vi "run.vi"(8 "error in (no error)":errorcluster, 11 "GenericScanMode in":refnum<class "GenericImagingMode.lvclass">) -> (0 "error out":errorcluster, 3 "GenericScanMode out":refnum<class "GenericImagingMode.lvclass">)   [LabVIEW 2010, in "GenericImagingMode.lvclass"]
uses:
  GenericImagingMode.lvclass
  common/classes/GenericToplevelComponent/GenericToplevelComponent/common_trigger_enum.ctl
  common/classes/ErrorController/ErrorController/class_data.vi
  common/classes/ErrorController/ErrorController/ErrorController.lvclass
  common/classes/GenericToplevelComponent/GenericToplevelComponent/GenericToplevelComponent.lvclass
panel:
  # "Functionality not available..."
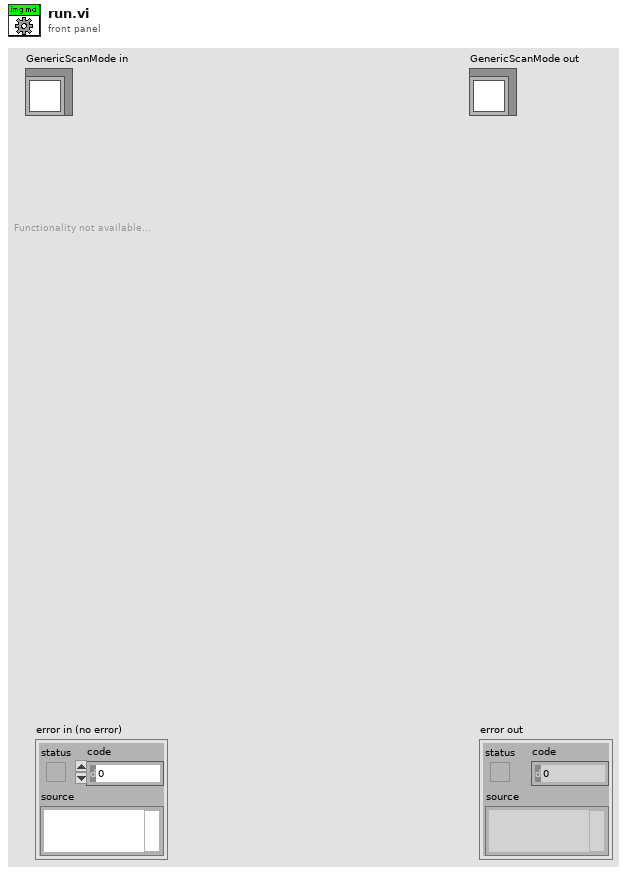
[diagram p1: front panel]
types:
  T1 = typedef "GenericToplevelComponent.lvclass/common_trigger_enum.ctl" = enum16{"NULL", "initialise", "terminate", "fetch command", "fetch data", "attach observer", "register as observer", "detach observer", "acknowledge", "start", "stop", "sweep started", "sweep finished", "experiment started", "experiment stopped"}
  T2 = typedef "main_trigger_enum.ctl" = enum16{"NULL", "initialise", "terminate", "start", "stop", "change objective", "change experimentController", "change imagingMode", "save notebook", "started saving", "finished saving", "expCtr ready", "expCtr missing", "imgMd ready", "imgMd missing", "scanHd ready", "scanHd missing", "DAQ ready", "DAQ missing", "imgAsm ready", "imgAsm missing", "dataColl ready", "dataColl missing", "display ready", "display missing", "analysr ready", "analysr missing", "instrmnt ready", "instrmnt missing", "stimltr ready", "stimltr missing", "stage ready", "stage missing"}
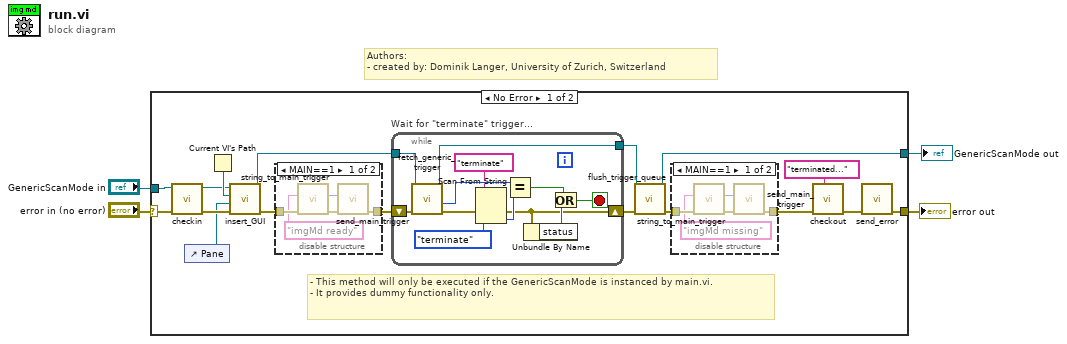
[diagram p0: block diagram]
diagram:
  # "Authors: \n- created by: Dominik Langer, University of Zurich, Switzerland"
  n1 = case shown="No Error" "error in (no error)" {
    selector: "error in (no error)" -> [w12 w47]
    tunnel: [w20 w47] -> w2
    tunnel: [w18 w46] -> w1
    tunnel: "GenericScanMode in" -> [w11 w46]
    frame No Error {
      # "- This method will only be executed if the GenericScanMode is instanced by main.vi.\n- It provides dummy functionality only."
      n2 = call-dynamic "checkin.vi"("error in (no error)"=w12, "GenericScanMode in"=w11) -> ("error out"=w10:errorcluster, "GenericScanMode out"=w9:refnum<class "GenericImagingMode.lvclass">)  [unwired: 8 in]
      n3 = control-ref of="Pane"() -> (w5:refnum<vi>)
      n4 = Current VI's Path() -> (path=w21:path)
      n5 = call-dynamic "insert_GUI.vi"("error in (no error)"=w10, "Pane"=w5, "VI path"=w21, "GenericComponent in"=w9) -> ("error out"=w14:errorcluster, "GenericComponent out"=w16:refnum<class "GenericImagingMode.lvclass">)  [unwired: 6 in]
      n6 = disable-structure shown="MAIN==1" {
        disable-tunnel: [w26 w27] -> w13
        disable-tunnel: w14 -> [w25 w27]
        frame condition #0 {
          n7 = call "string_to_main_trigger.vi"("error in (no error)"=w25, "trigger string"="imgMd ready") -> ("error out"=w24:errorcluster, "main trigger"=w23:T2)  [unwired: 8 in]
          n8 = call "send_main_trigger.vi"("error in (no error)"=w24, "trigger"=w23) -> ("error out"=w26:errorcluster)  [unwired: 9 in]
        }
        frame condition #1 (active) {
        }
      }
      n9 = while "Wait for \"terminate\" trigger..." {
        tunnel: w16 -> [w42]
        tunnel: [w40] -> w17
        shift-right: [w36] -> w19
        shift-left: w13 -> [w43]
        stop <- w44 stop-if-true
        n10 = call-dynamic "fetch_generic_trigger.vi"("error in (no error)"=w43, "GenericToplevelComponent in"=w42) -> ("error out"=w37:errorcluster, "common trigger"=w35:T1, "GenericToplevelComponent out"=w40:refnum<class "GenericImagingMode.lvclass">)  [unwired: 3 in, 4 out]
        n11 = Scan From String(input string="terminate", error in=w37, default 1=common_trigger_enum."terminate" ("x")) -> (error out=w36:errorcluster, output 1=w38:T1)  [unwired: 2 in, 2 out]
        n12 = Equal?(x=w35, y=w38) -> (x = y?=w41:bool)
        n13 = Unbundle By Name(w36) -> ("status"=w45:bool)
        n14 = Or(x=w41, y=w45) -> (x .or. y?=w44:bool)
      }
      n15 = call-dynamic "flush_trigger_queue.vi"("error in (no error)"=w19, "GenericToplevelComponent in"=w17) -> ("error out"=w15:errorcluster, "GenericToplevelComponent out"=w18:refnum<class "GenericImagingMode.lvclass">)  [unwired: 8 in]
      n16 = disable-structure shown="MAIN==1" {
        disable-tunnel: [w32 w33] -> w8
        disable-tunnel: w15 -> [w31 w33]
        frame condition #0 {
          n17 = call "string_to_main_trigger.vi"("error in (no error)"=w31, "trigger string"="imgMd missing") -> ("error out"=w30:errorcluster, "main trigger"=w29:T2)  [unwired: 8 in]
          n18 = call "send_main_trigger.vi"("error in (no error)"=w30, "trigger"=w29) -> ("error out"=w32:errorcluster)  [unwired: 9 in]
        }
        frame condition #1 (active) {
        }
      }
      n19 = call "checkout.vi"("locked by?"="terminated...", "error in (no error)"=w8) -> ("error out"=w6:errorcluster)  [unwired: 8 in, 1 out]
      n20 = call "send_error.vi"("error in (no error)"=w6) -> ("error out"=w20:errorcluster)  [unwired: 10 in]
    }
    frame Error {
    }
  }
  "error out" <- w2
  "GenericScanMode out" <- w1
